vi "test-new-clock.vi"() -> ()   [LabVIEW 2019]
panel:
  out "OS Clock":dbl format="%35.6f"
  out "Waveform Chart":cluster{"FPGA_Time_Seconds":dbl, dbl, dbl}(graph)
  out "Error Count":i32
  out "Loop Count":i32
  out "FPGA Clock":dbl format="%35.6f"
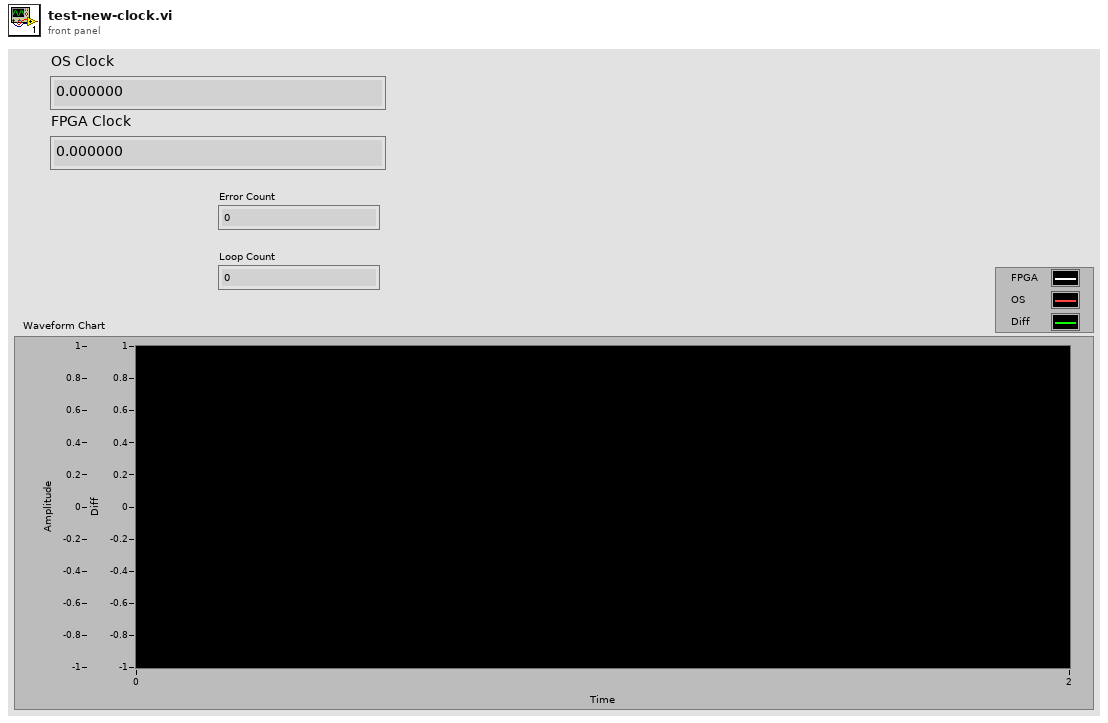
[diagram p1: front panel]
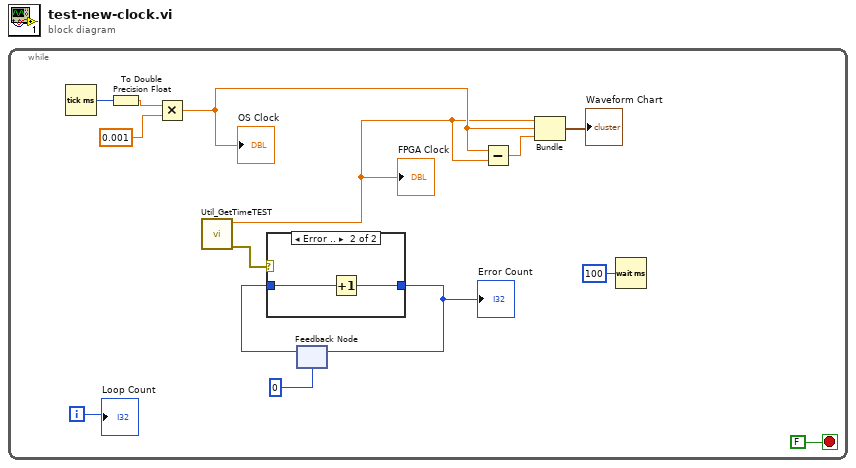
[diagram p0: block diagram]
diagram:
  n1 = while {
    i -> [w13]
    stop <- FALSE stop-if-true
    n2 = Tick Count (ms)() -> (millisecond timer value=w6:u32)
    n3 = To Double Precision Float(number=w6) -> (double precision float=w5:dbl)
    n4 = Multiply(x=w5, y=0.001) -> (x*y=w3:dbl)
    "OS Clock" <- w3
    n5 = call "Util_GetTimeTEST.vi"() -> ("error out"=w11:errorcluster, "FPGA_Time_Seconds"=w2:dbl)  [unwired: 10 in]
    "FPGA Clock" <- w2
    n6 = feedback #1(0) -> (w10:i32)
    n7 = case shown="Error .." w11 {
      tunnel: w10 -> [w15 w16]
      tunnel: [w15 w17] -> w9
      frame No Error {
      }
      frame Error {
        n8 = Increment(x=w16) -> (x+1=w17:i32)
      }
    }
    "Error Count" <- w9
    n9 = feedback-in #1(w9) -> ()
    n10 = Subtract(x=w3, y=w2) -> (x-y=w1:dbl)
    n11 = Bundle("FPGA_Time_Seconds"=w2, w3, w1) -> (→"Waveform Chart":cluster{"FPGA_Time_Seconds":dbl, dbl, dbl})  [unwired: 1 in]
    n12 = Wait (ms)(milliseconds to wait=u32 100) -> ()  [unwired: 1 out]
    "Loop Count" <- w13
  }
